vi "AlliGator Compute Phasor Plot.vi"(8 "error in (no error)":errorcluster, 9 "Compute Phasor Plot (F)":bool, 10 "Pre-processed Sum Image (V x H)":sgl[][](array[numeric]), 11 "Pixel Phasors Array":csg[][](array[numeric])) -> (0 "error out":errorcluster, 1 "elapsed (relative) seconds":dbl, 2 "Phasor Plot Reference Points":T1, 3 "Phasor Plot":sgl[][](array[numeric]))   [LabVIEW 2021, in "AlliGator Phasor Plot.lvlib"]
uses:
  AlliGator Phasor Plot.lvlib
  Phasor Ratio/AlliGator Phasor Plot Reference Points.ctl
  Globals, Variables, Constants/AlliGator Variables List.ctl
  Settings/AlliGator Settings List.ctl
  AlliGator Phasor Plot Size.ctl
  f53e779f-ac1e-4712-8ab8-863940e9679a.vi
  Variant/Variant to Data/Variant to Boolean.vi
  Globals, Variables, Constants/AlliGator Globals, Variables & Constants.lvlib
  Phasor Ratio/AlliGator Phasor Ratio.lvlib
  Settings/AlliGator Settings.lvlib
  Time/Time.lvlib
  Variant/Variant to Data/Variant to Data.lvlib
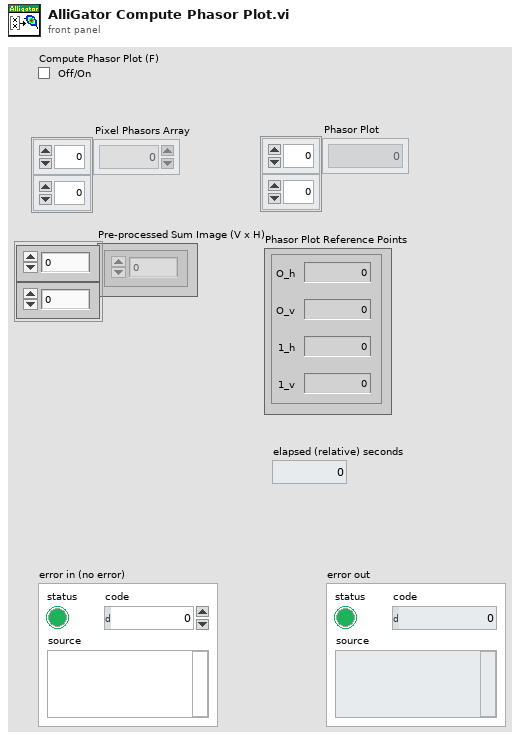
[diagram p1: front panel]
types:
  T1 = typedef "AlliGator Phasor Ratio.lvlib/AlliGator Phasor Plot Reference Points.ctl" = cluster{"O_h":dbl, "O_v":dbl, "1_h":dbl, "1_v":dbl}
  T2 = typedef "AlliGator Settings.lvlib/AlliGator Settings List.ctl" = enum16{"GUI:Visible Settings Tab", "GUI:Last Run Version", "Source Image:Use Image Histogram for Contrast", "Source Image:Low Count Pixels Rejection Options", "Source Image:High Count Pixels Rejection Options", "Source Image:Use Image Brightness", "Source Image:Blend Overlay with Image Background", "Source Image:Use Fixed ROI Diameter", "Source Image:ROI Diameter", "Source Image:ROI Center Color", "Source Image:Peak Threshold", "Source Image:Intensity Threshold", "Source Image:Image Binning Options", "Source Image:Image Smoothing Options", "Source Image:Image Histogram Active", "Source Image:Invert Binary Mask", "Source Image:Hot Pixel Removal", "Source Image:Overlay Analyzed ROI Center", "Source Image:Auto-Adjust Contrast", "Source Image:Histogram Lower Percentile", "Source Image:Histogram Upper Percentile", "Source Image:Save Source Image", "Source Image:Scale Bar Options", "Source Image:Image Resolution (Pixel Size)", "Source Image:Flatfield Correction", "Source Image:Show Dead Left Columns Correction", "Source Image:Dead Left Columns Correction", "Source Image:Image Pre-Processing Operations Order", "Source Image:Overlay ROI Median", "Source Image:Median Overlay Color", "Data Information:Gate Width", "Data Information:Nanotime Gate Separation", "Data Information:Macrotime Gate Separation", "Data Information:Gate Step", "Data Information:# Gates", "Data Information:Gate Image Exposure", "Data Information:Gate Image Integration", "Data Information:Gates to Skip", "Data Information:Gates to Keep", "Data Information:Define Gates to", "Data Information:Channel Name", "Data Information:Available Channel Names", "Data Information:Channel Arithmetic", "Data Information:Background File Subtraction", "Data Information:Background File", "Data Information:Background Scaling Factor", "Data Information:Background Pile-up Correction", "Data Information:Background Pixel Well Capacity", "Data Information:Laser Period", "Data Information:SYNC Period", "Data Information:Pile-up Correction", "Data Information:Pixel Well Capacity", "Data Information:Dataset Scaling Factor", "Fluorescence Decay_Decay Pre-Processing:Reverse Gates", "Fluorescence Decay_Decay Pre-Processing:Verbose Decay Pre-Processing", "Fluorescence Decay_Decay Pre-Processing:Use Decay Pre-Processing", "Fluorescence Decay_Decay Pre-Processing:Background Subtraction", "Fluorescence Decay_Decay Pre-Processing:Background Definition Range", "Fluorescence Decay_Decay Pre-Processing:Baseline Subtraction Method", "Fluorescence Decay_Decay Pre-Processing:Decay Pre-Processing Operations Order", "Fluorescence Decay_Decay Pre-Processing:Smoothing Parameter", "Fluorescence Decay_Decay Pre-Processing:Shift Decay", "Fluorescence Decay_Decay Pre-Processing:Decay Shift Parameters", "Fluorescence Decay_Decay Pre-Processing:Fold Decay", "Fluorescence Decay_Decay Pre-Processing:# Folds", "Fluorescence Decay_Decay Pre-Processing:1-Normalize Decay", "Fluorescence Decay_Decay Pre-Processing:[0-1]-Normalize Decay", "Fluorescence Decay_Decay Pre-Processing:Smoothen Decay", "Fluorescence Decay_Decay Pre-Processing:Extrapolate Decay", "Fluorescence Decay_Decay Pre-Processing:Use Periodicity", "Fluorescence Decay_Decay Pre-Processing:Use Cursors", "Fluorescence Decay_Decay Pre-Processing:Tail Fraction", "Fluorescence Decay_Decay Pre-Processing:Head Fraction", "Fluorescence Decay_Decay Pre-Processing:Additional Points", "Fluorescence Decay_Decay Pre-Processing:Straighten Decay", "Fluorescence Decay_Decay Pre-Processing:Constant Background", "Fluorescence Decay_Decay Pre-Processing:Pixel-Normalize Decay", "Fluorescence Decay_Advanced Analysis:Extract IRF instead of Decay", "Fluorescence Decay_Advanced Analysis:IRF Extraction Options", "Fluorescence Decay_Advanced Analysis:IRF Optimization Options", "Fluorescence Decay_Advanced Analysis:Square Pulse Options", "Fluorescence Decay_Advanced Analysis:IRF Order", "Fluorescence Decay_Advanced Analysis:IRF Time Constants", "Fluorescence Decay_Advanced Analysis:Wavelet Analysis Options", "Fluorescence Decay_Advanced Analysis:Average Lifetime Options", "Fluorescence Decay_Fit Options:Fit Options", "Fluorescence Decay_Fit Options:Use Legacy Fitting Approach", "Fluorescence Decay_Fit Options:Use Data Information Laser Period", "Fluorescence Decay_Fit Parameters:Displayed Fit Parameters", "Fluorescence Decay_Fit Parameters:Fit Parameter Constraints", "Fluorescence Decay_Fit Parameters:Export Tabulated Results", "Fluorescence Decay_Fit Parameters:MLE Baseline Offset Type", "Fluorescence Decay_Fit Parameters:MLE Baseline Offset", "Fluorescence Decay_Fit Parameters:Guess Parameter Names", "Fluorescence Decay_Fit Parameters:Guess Parameter Values", "Fluorescence Decay_Fit Parameters:Guess Parameters Options", "Fluorescence Decay_Fit Parameters:Optimal Offset Selection Criterion", "Fluorescence Decay_Styles:Show Last Decay Only", "Fluorescence Decay_Styles:Decay Graph Color Array", "Fluorescence Decay:Decay Graph Active", "Fluorescence Decay Statistics:Min Peak Value", "Fluorescence Decay Statistics:Reject Low Decay Peak Pixels", "Fluorescence Decay Statistics:Reject High Decay Peak Pixels", "Fluorescence Decay Statistics:Max Peak Value", "Time Traces:Use File Timestamp", "Time Traces:Time Step", "Time Traces:Use Intensity Correction File", "Time Traces:Intensity Correction File", "Phasor Plot:Phasor Plot Smoothing Options", "Phasor Plot:Phasor Plot Size", "Phasor Plot:Phasor Plot Graphics Options", "Phasor Plot:Cumulative Phasor Plot", "Phasor Plot:Use Phasor Brightness", "Phasor Plot:Blend Overlay with Phasor Background", "Phasor Plot:Save Phasor Plot", "Phasor Plot:Show References", "Phasor Plot:Phasor Ratio Decay Range", "Phasor Plot:Exponential Fading", "Phasor Plot:Phasor Ratio Reference Colors", "Phasor Plot:Reference Radius", "Phasor Plot:Show Color Map Vertices", "Phasor Plot:Phasor Plot Active", "Phasor Plot:Phasor Ratio Color Map Type", "Phasor Plot:Phasor Ratio Color Map", "Phasor Plot:Phasor Ratio Display Range", "Phasor Plot:Selected Image ROI(s)", "Phasor Plot:All Image ROIs", "Phasor Plot:Selected Phasor Plot ROI(s)", "Phasor Plot:All Phasor Plot ROIs", "Phasor Plot:Phasor Ratio Color-Coded Quantity", "Phasor Plot:Store Phasor Harmonics", "Phasor Plot:Draw Reference Segment", "Phasor Plot:User-Defined Quantity", "Phasor Plot:Color Scale High Color", "Phasor Plot:Color Scale Low Color", "Phasor Plot:Intensity-weighted Phasor Plot", "Phasor Graph:Phasor Frequency", "Phasor Graph:Phasor Ratio Type", "Phasor Graph:Pixel-level Phasor Computation", "Phasor Graph:Save Phasor Graph", "Phasor Graph:Phasor Graph Active", "Phasor Graph:Phasor SDV Options", "Phasor Calibration:Use Backup Calibration if needed", "Phasor Graph:Define Shortest Lifetime as", "Phasor Calibration:Backup Calibration Type", "Phasor Calibration:Calibration Type", "Phasor Calibration:Calibration Lifetime", "Phasor Calibration:Calibration Map Algorithm", "Single-Exponential Phasor Locus (SEPL):Gate Parameters", "Single-Exponential Phasor Locus (SEPL):User-defined Gate", "Single-Exponential Phasor Locus (SEPL):User-defined IRF", "Single-Exponential Phasor Locus (SEPL):Phasor Parameters", "Single-Exponential Phasor Locus (SEPL):Decay & IRF Parameters", "Single-Exponential Phasor Locus (SEPL):Display Parameters", "Lifetime Analysis:Decay Analysis Parameters", "Lifetime Analysis:Lifetime Map Active", "Plugins:Python Settings", "Miscellaneous:Verbose Mode", "Miscellaneous:Beep after Script", "Miscellaneous:Saved Image File Format", "Miscellaneous:Exported Gate Image Settings", "Miscellaneous:Include Loading in Timing", "Miscellaneous:Verbose Settings Mode", "Miscellaneous:Histogram Options", "Miscellaneous:Beep on Error", "Miscellaneous:# Logical Processors Used", "Miscellaneous:ROI Description Max Characters", "Miscellaneous:Verbose Error Mode", "Miscellaneous:Transparent Mask Color"}
  T3 = typedef "AlliGator Phasor Plot.lvlib/AlliGator Phasor Plot Size.ctl" = cluster{"H":i32, "V":i32, "Margin":dbl}
  T4 = typedef "AlliGator Globals, Variables & Constants.lvlib/AlliGator Variables List.ctl" = enum16{"---- GUI ----", "GUI:Initialization Status", "GUI:State Indicators Refnum", "GUI:Original AlliGator Menu Items", "GUI:Current Action Loop State", "GUI:Script in progress", "GUI:Playback", "GUI:Loop Playback", "GUI:Search ROI Used", "GUI:Search ROI", "Decay Graph Max Legend Size", "Intensity Graph Max Legend Size", "Decay Statistics Graph Max Legend Size", "Phasor Graph Max Legend Size", "Phasor Ratio Graph Max Legend Size", "Lifetime Graph Max Legend Size", "---- Files ----", "Files:Export Dataset Frames as Individual Files", "Files:Show Batch Export Help Balloons", "Files:Frames in Dataset", "Files:ptu File Frame Start Indices", "Files:Current Frame in Dataset", "Files:Current Frame Timestamp", "Files:Dataset Loaded", "Files:Dataset Metadata", "Files:Dataset Channel", "Files:Dataset Data Description", "Files:Background Dataset Metadata", "Files:Background Dataset Channel", "Files:Background Dataset Data Description", "Files:Background File Subtraction", "Files:Background File Path", "Files:Background File Pile-up Correction", "Files:Background File Pixel Well Capacity", "Files:Background File Scaling Factor", "Files:Current Dataset Load Settings", "Files:Dataset Path", "Files:ICCD-specific Information", "Files:Macrotime Gate Separation", "------ Python Plugins ------", "Python Plugins:Information", "Python Plugins:Python Session", "Python Plugins:Valid Python Session?", "---- Source Image ----", "Source Image:ROIs", "Source Image:Current ROI", "Source Image:ROI Event Refnum", "X_Source Image:Display Range", "X_Source Image:Palette Information", "X_Source Image:Type of Displayed Image", "X_Time Gate Slider", "Source Image:Palette List", "Source Image:Scale", "Source Image:ROI Overlay Color", "Source Image:Overlay to Erase", "Source Image:Is Displayed Image Accumulated", "Source Image:White Light Image Modified", "Source Image:Mask Image Modified", "---- Image Profile Window ----", "Image Profile:Window Event Refnum", "Image Profile:IntensityType", "Image Profile:Intensity Average Type", "Image Profile:Intensity-weighted SDV", "Image Profile:Box Profile Type", "Image Profile:Window Open", "Image Profile:Plotted Fit Parameter", "------ Phasor Graph -------", "Phasor Graph:Show Line", "---- Phasor Plot ---", "Phasor Plot:Parameters Changed", "Phasor Plot:FLI Dataset Modified since last Calculation", "Phasor Harmonics Data", "Selected Phasor Harmonics", "Phasor Harmonic Manager Event Refnum", "Phasor Plot:ROIs", "Phasor Plot:Current ROI", "Phasor Plot:ROI Event Refnum", "Phasor Plot:Image Reference Points", "Phasor Plot:Computed", "Phasor Plot:Palette Information", "Phasor Plot:Palette List", "Phasor Plot:Phasor Ratio Palette Information", "Phasor Plot:Phasor Ratio Palette List", "Phasor Plot:Image Scale", "Phasor Plot:Image Overlay to Erase", "Phasor Plot:Image Elements to Update", "Phasor Plot:Current Calculation Parameters", "Phasor Plot:Current Calibration Options", "Phasor Plot:Reset Cumulated Phasor Plot", "Phasor Plot:Reference 1", "Phasor Plot:Lifetime Reference 1", "Phasor Plot:Reference 1 Frequency", "Phasor Plot:Reference 2", "Phasor Plot:Lifetime Reference 2", "Phasor Plot:Reference 2 Frequency", "---- Decay Analysis ----", "Number of Selected Decays to Fit", "LS Fit Results", "LAR Fit Results", "BS Fit Results", "Last Decay Max - Min", "Best Fit Parameters", "Best Fit Parameter Names", "Actual Size X", "Actual Size Y", "Binning X", "Binning Y", "Actual # Gates", "Dataset Number", "Gates to...", "Gates Skipped", "Gates to keep", "Gate Step", "Gate Separation", "Reversed Gates", "Pile-up Correction", "Pixel Well Capacity", "Background Subtracted", "Background Subtraction Method", "Background Definition Range", "Background File (deprecated)", "Number of Dataset Accumulated", "Array of Accumulated Dataset Paths", "Do Averaged Datasets", "Destination File Path", "Process Plot Target", "Use 1/D as Phasor Frequency", "---- Decay Fit Parameter Map -----", "Decay Fit Parameter Map:Palette Information", "Decay Fit Parameter Map:Palette List", "Decay Fit Parameter Map:X Resolution", "Decay Fit Parameter Map:Y Resolution", "---- Parameter Map ----", "Parameter Map:Palette Information", "Parameter Map:Palette List", "------- Local Decay Window ---------", "Local Decay Graph Window:Event Refnum", "Local Decay Graph Window:Use normalized IRF for convolution", "----- Miscellaneous ----", "Misc:Skippable Dialog Windows Status"}
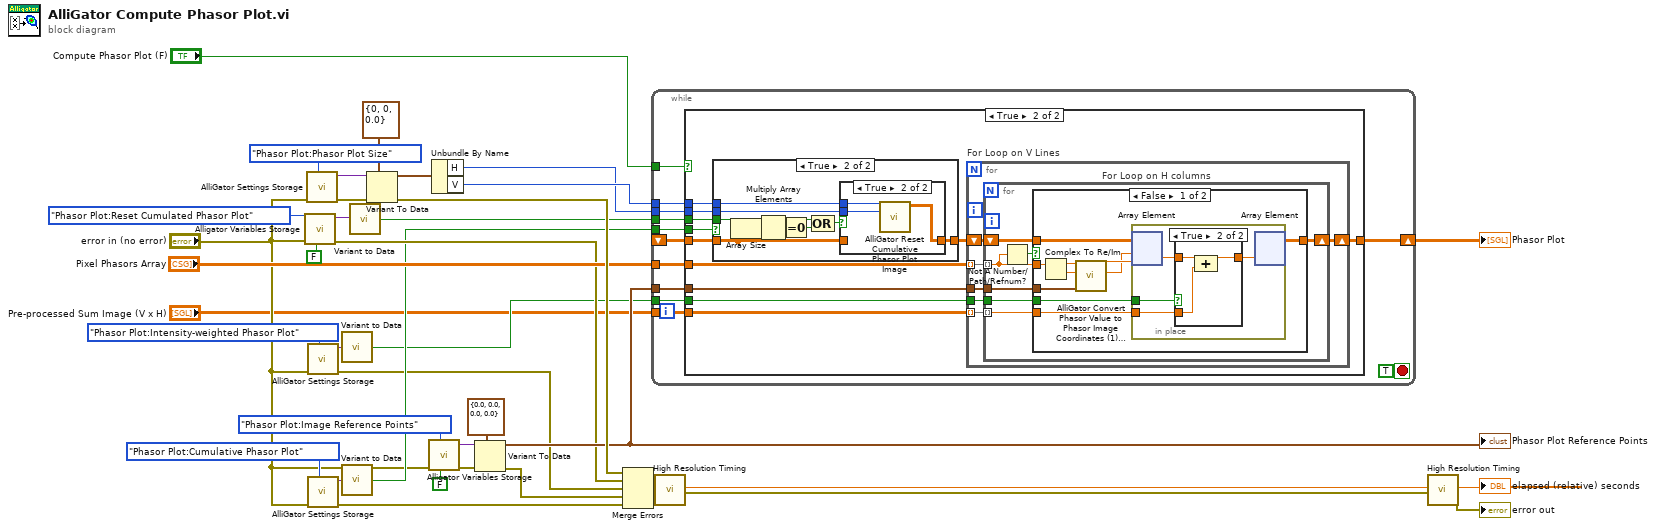
[diagram p0: block diagram]
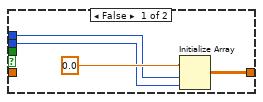
[diagram p3: hidden frame]
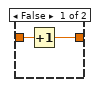
[diagram p5: hidden frame]
diagram:
  n1 = call "Alligator Variables Storage.vi"("Get(F)/Set"=FALSE, "AlliGator Variable"=AlliGator_Variables_List."Phasor Plot:Reset Cumulated Phasor Plot" ("Alligator Variable"), "Error In"="error in (no error)") -> ("Error Out"=w22:errorcluster, "Data out"=w13:variant)  [unwired: 6 in, 1 out]
  n2 = call "AlliGator Settings Storage.vi"("AlliGator Settings List"=AlliGator_Settings_List."Phasor Plot:Phasor Plot Size", "Error In"="error in (no error)") -> ("Error Out"=w33:errorcluster, "Variant Data out"=w31:variant)  [unwired: 8 in]
  n3 = call "AlliGator Settings Storage.vi"("AlliGator Settings List"=AlliGator_Settings_List."Phasor Plot:Intensity-weighted Phasor Plot", "Error In"="error in (no error)") -> ("Error Out"=w4:errorcluster, "Variant Data out"=w6:variant)  [unwired: 8 in]
  n4 = call "AlliGator Settings Storage.vi"("AlliGator Settings List"=AlliGator_Settings_List."Phasor Plot:Cumulative Phasor Plot", "Error In"="error in (no error)") -> ("Error Out"=w24:errorcluster, "Variant Data out"=w18:variant)  [unwired: 8 in]
  n5 = call-poly "Variant to Data.vi"("Variant"=w6) -> ("Value"=w3:bool)  [unwired: 8 in]
  n6 = call-poly "Variant to Data.vi"("Variant"=w18) -> ("Value"=w10:bool)  [unwired: 8 in]
  n7 = call-poly "Variant to Data.vi"("Variant"=w13) -> ("Value"=w16:bool)  [unwired: 8 in]
  n8 = Variant To Data(error in=w33, type=T3 {"H"=0, "V"=0, "Margin"=0.0} ("Phasor Plot Size"), Variant=w31) -> (data=w36:T3, error out=w34:errorcluster)
  n9 = call "Alligator Variables Storage.vi"("Get(F)/Set"=FALSE, "AlliGator Variable"=AlliGator_Variables_List."Phasor Plot:Image Reference Points" ("Alligator Variable"), "Error In"="error in (no error)") -> ("Error Out"=w9:errorcluster, "Data out"=w7:variant)  [unwired: 6 in, 1 out]
  n10 = Unbundle By Name(w36) -> ("H"=w37:i32, "V"=w38:i32)
  n11 = Variant To Data(error in=w9, type=T1 {"O_h"=0.0, "O_v"=0.0, "1_h"=0.0, "1_v"=0.0} ("Phasor Plot Reference Points"), Variant=w7) -> (data=w29:T1, error out=w23:errorcluster)
  "Phasor Plot Reference Points" <- w29
  n12 = Merge Errors(w34, w22, w4, w23, w24) -> (w21:errorcluster)
  n13 = while {
    tunnel: "Pixel Phasors Array" -> [w50]
    tunnel: w29 -> [w49]
    tunnel: w38 -> [w47]
    tunnel: w37 -> [w46]
    shift-right: [w48] -> w25
    shift-left: _ -> [w44]
    tunnel: w10 -> [w45]
    tunnel: w16 -> [w42]
    tunnel: "Compute Phasor Plot (F)" -> [w41]
    tunnel: w3 -> [w40]
    tunnel: "Pre-processed Sum Image (V x H)" -> [w39]
    stop <- TRUE stop-if-true
    n14 = case shown="True" w41 {
      tunnel: w50 -> [_ w62]
      tunnel: w49 -> [_ w61]
      tunnel: [w51 w59] -> w48
      tunnel: w47 -> [_ w58]
      tunnel: w46 -> [_ w57]
      tunnel: w45 -> [_ w56]
      tunnel: w44 -> [w51 w55]
      tunnel: w42 -> [_ w54]
      tunnel: w40 -> [_ w53]
      tunnel: w39 -> [_ w52]
      frame False {
      }
      frame True {
        n15 = case shown="True" w56 {
          tunnel: [w66 w74] -> w60
          tunnel: w58 -> [w64 w73]
          tunnel: w57 -> [w63 w72]
          tunnel: w55 -> [_ w71]
          tunnel: w54 -> [_ w75]
          frame False {
            n16 = Initialize Array(sgl 0.0, w64, w63) -> (w66:sgl[][])
          }
          frame True {
            n17 = Array Size(array=w71) -> (size(s)=w70:i32[])
            n18 = Multiply Array Elements(1:w70) -> (0:w69:i32)
            n19 = Equal To 0?(x=w69) -> (x = 0?=w67:bool)
            n20 = Compound Arithmetic op=OR(w75, w67) -> (w68:bool)
            n21 = case shown="True" w68 {
              tunnel: w71 -> [w76 _]
              tunnel: [w76 w77] -> w74
              tunnel: w73 -> [_ w79]
              tunnel: w72 -> [_ w78]
              frame False {
              }
              frame True {
                n22 = call "AlliGator Reset Cumulative Phasor Plot Image.vi"("X Resolution"=w78, "Y Resolution"=w79) -> ("Array"=w77:sgl[][])  [unwired: 9 in]
              }
            }
          }
        }
        n23 = for "For Loop on V Lines" {
          tunnel: w62 -> [w85] mode=indexing
          tunnel: w61 -> [w84]
          shift-right: [w82] -> w59
          shift-left: w60 -> [w83]
          tunnel: w53 -> [w81]
          tunnel: w52 -> [w80] mode=indexing
          n24 = for "For Loop on H columns" {
            tunnel: w85 -> [w89] mode=indexing
            tunnel: w84 -> [w92]
            shift-right: [w90] -> w82
            shift-left: w83 -> [w91]
            tunnel: w81 -> [w87]
            tunnel: w80 -> [w86] mode=indexing
            n25 = Not A Number/Path/Refnum?(number/path/refnum=w89) -> (NaN/Path/Refnum?=w88:bool)
            n26 = case shown="False" w88 {
              tunnel: w92 -> [w102 _]
              tunnel: w91 -> [w99 w112]
              tunnel: [w98 w112] -> w90
              tunnel: w89 -> [w95 _]
              tunnel: w87 -> [w94 _]
              tunnel: w86 -> [w93 _]
              frame False {
                n27 = Complex To Re/Im(x + iy=w95) -> (x=w101:sgl, y=w100:sgl)
                n28 = call "AlliGator Convert Phasor Value to Phasor Image Coordinates (1).vim"("Phasor Plot Reference Points"=w102, "Phasor s"=w100, "Phasor g"=w101) -> ("Phasor Plot y"=w96:dbl, "Phasor Plot x"=w97:dbl)  [unwired: 7 in]
                n29 = in-place {
                  in-place-border: w94 -> [w104]
                  in-place-border: w93 -> [w103]
                  n30 = in-place-array #1(w99, w96, w97) -> (w106:sgl)
                  n31 = case shown="True" w104 {
                    tunnel: w106 -> [w108 w111]
                    tunnel: [w107 w110] -> w105
                    tunnel: w103 -> [_ w109]
                    frame False {
                      n32 = Increment(x=w108) -> (x+1=w107:sgl)
                    }
                    frame True {
                      n33 = Compound Arithmetic op=ADD(w111, w109) -> (w110:sgl)
                    }
                  }
                  n34 = in-place-array #1(w105) -> (w98:sgl[][])  [unwired: 2 out]
                }
              }
              frame True {
              }
            }
          }
        }
      }
    }
  }
  "Phasor Plot" <- w25
  n35 = call "High Resolution Timing.vi"("Error In"=w21) -> ("elapsed (relative) seconds"=w19:dbl, "Error Out"=w30:errorcluster)  [unwired: 16 in, 1 out]
  n36 = call "High Resolution Timing.vi"("relative seconds (NaN)"=w19, "Error In"=w30) -> ("elapsed (relative) seconds"=→"elapsed (relative) seconds":dbl, "Error Out"=→"error out":errorcluster)  [unwired: 15 in, 1 out]
